vi "2DGraphSetup.vi"(8 "error in (no error)":errorcluster caption="entrée d'erreur (pas d'erreur)", 11 "Interface en entrée":refnum<class "Interface.lvclass"> caption="DNL_LabVIEW Object in") -> (0 "error out":errorcluster caption="sortie d'erreur", 3 "Interface en sortie":refnum<class "Interface.lvclass"> caption="DNL_LabVIEW Object out")   [LabVIEW 2019, in "Interface.lvclass"]
uses:
  Interface.lvclass
  Interface.lvclass/Interface.ctl
  <userlib>/GenProg/ArrayTo1DString.vi
  Experiment Class/Experiment.lvclass
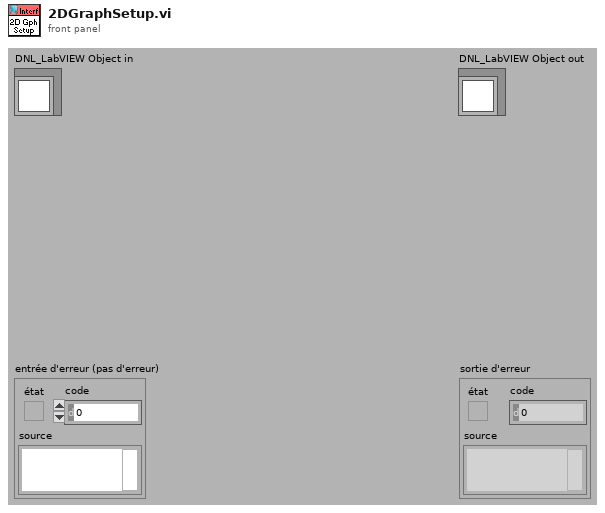
[diagram p1: front panel]
types:
  T1 = typedef "2DGraphSetup.ctl" = cluster{"ZDataIndex":i32, "XParIndex":i32, "YParIndex":i32, "FillLineFirst":bool, "2DGraphIndex":i32, "XParQ Ref":refnum<queue>, "YParQ Ref":refnum<queue>, "DataQRefs":refnum<queue>[], "CurveName":string, "XparInstrInd":i32, "YparInstrInd":i32, "Active":bool}
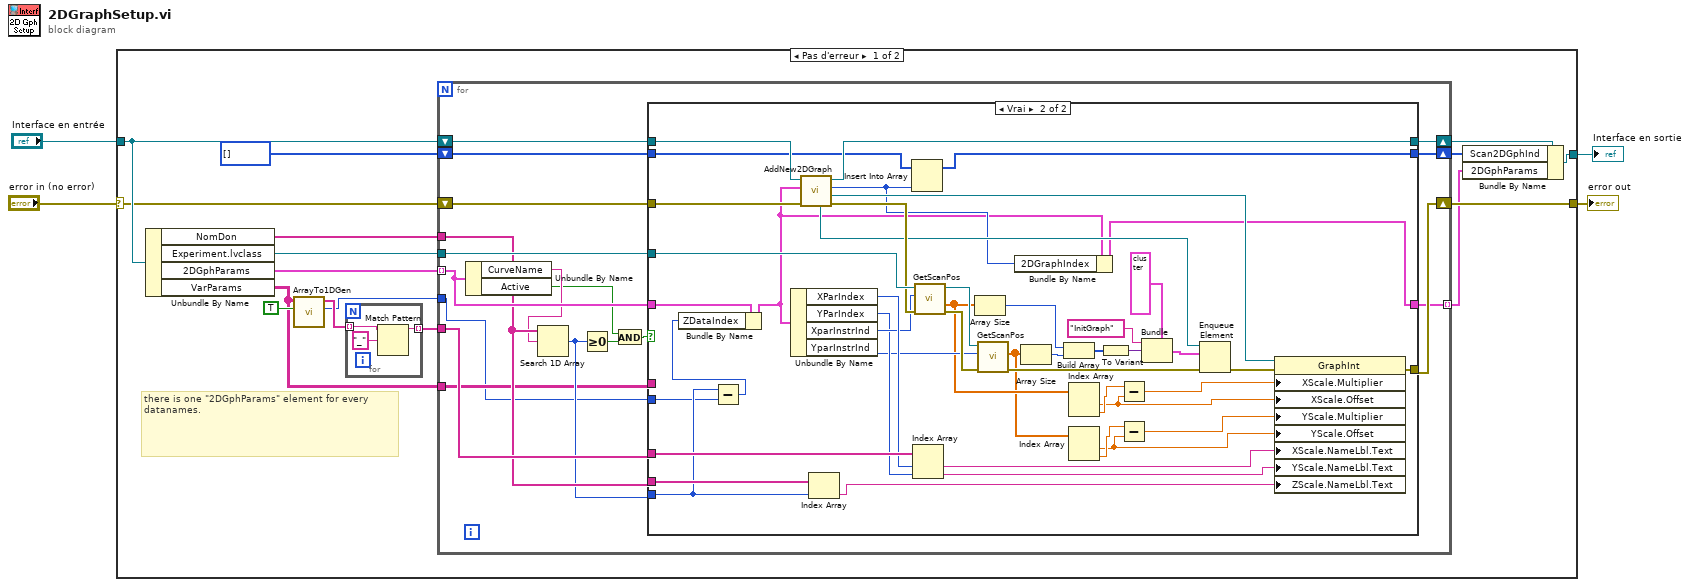
[diagram p0: block diagram]
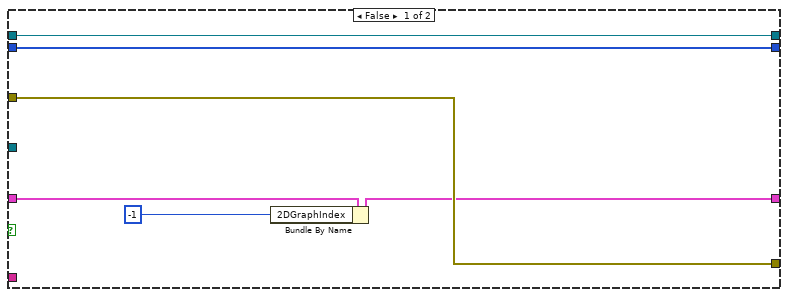
[diagram p2: hidden frame]
diagram:
  n1 = case shown="Pas d'erreur" "error in (no error)" {
    selector: "error in (no error)" -> [w14 w94]
    tunnel: [w12 w94] -> w3
    tunnel: [w17 w93] -> w1
    tunnel: "Interface en entrée" -> [w20 w93]
    frame No Error {
      # "there is one \"2DGphParams\" element for every datanames."
      n2 = Unbundle By Name(w20) -> ("NomDon"=w9:string[], "Experiment.lvclass"=w19:refnum<class "Experiment.lvclass">, "2DGphParams"=w13:T1[], "VarParams"=w7:string[][])
      n3 = call-poly <userlib>:"ArrayTo1DGen.vi"("DelArrEnd"=TRUE, "tableau"=w7) -> ("Size"=w5:i32, "Array Out"=w8:string[])  [unwired: 7 in, 1 out]
      n4 = for {
        tunnel: w8 -> [w23] mode=indexing
        tunnel: [w22] -> w10 mode=indexing
        n5 = Match Pattern(string=w23, regular expression="_" ("expression régulière")) -> (before substring=w22:string)  [unwired: 1 in, 3 out]
      }
      n6 = for {
        tunnel: w13 -> [w41] mode=indexing
        shift-right: [w39] -> w18
        shift-left: w20 -> [w40]
        tunnel: w19 -> [w38]
        shift-right: [w37] -> w16
        shift-left: i32[] [] -> [w36]
        shift-right: [w35] -> w12
        shift-left: w14 -> [w34]
        tunnel: w10 -> [w33]
        tunnel: w9 -> [w32]
        tunnel: w7 -> [w29]
        tunnel: [w25] -> w6 mode=indexing
        tunnel: w5 -> [w24]
        n7 = Unbundle By Name(w41) -> ("CurveName"=w31:string, "Active"=w26:bool)
        n8 = Search 1D Array(1D array=w32, element=w31) -> (index of element=w30:i32)  [unwired: 1 in]
        n9 = Greater Or Equal To 0?(x=w30) -> (x >= 0?=w27:bool)
        n10 = And(x=w26, y=w27) -> (x .and. y?=w28:bool)
        n11 = case shown="Vrai" w28 {
          tunnel: w41 -> [w44 w54]
          tunnel: w40 -> [w47 w92]
          tunnel: [w47 w91] -> w39
          tunnel: w38 -> [_ w88]
          tunnel: [w46 w90] -> w37
          tunnel: w36 -> [w46 w89]
          tunnel: [w45 w73] -> w35
          tunnel: w34 -> [w45 w72]
          tunnel: w33 -> [_ w69]
          tunnel: w32 -> [_ w65]
          tunnel: w30 -> [_ w50]
          tunnel: w29 -> [_ _]
          tunnel: [w43 w53] -> w25
          tunnel: w24 -> [_ w49]
          frame False {
            n12 = Bundle By Name(cluster=w44, "2DGraphIndex"=-1) -> (w43:T1)
          }
          frame True {
            n13 = Subtract(x=w50, y=w49) -> (x-y=w48:i32)
            n14 = Bundle By Name(cluster=w54, "ZDataIndex"=w48) -> (w51:T1)
            n15 = Unbundle By Name(w51) -> ("XParIndex"=w67:i32, "YParIndex"=w62:i32, "XparInstrInd"=w63:i32, "YparInstrInd"=w61:i32)
            n16 = call "AddNew2DGraph.vi"("error in (no error)"=w72, "2DGphParam"=w51, "Interface en entrée"=w92) -> ("error out"=w71:errorcluster, "Graph"=w87:refnum<vi>, "NewGraphInd"=w52:i32, "Interface en sortie"=w91:refnum<class "Interface.lvclass">, "2DGraphQRef"=w70:refnum<queue>)  [unwired: 4 in]
            n17 = Index Array(array=w65, index=w50) -> (element=w64:string)
            n18 = Insert Into Array(array=w89, new element=w52) -> (w90:i32[])  [unwired: 1 in]
            n19 = Index Array(array=w69, index #1=w67, index #2=w62) -> (element #1=w68:string, element #2=w66:string)
            n20 = call "GetScanPos.vi"("error in (no error)"=w71, "ParIndex"=w63, "Experiment en entrée"=w88) -> ("error out"=w83:errorcluster, "ScanTable"=w56:dbl[], "Experiment en sortie"=w84:refnum<class "Experiment.lvclass">)  [unwired: 6 in]
            n21 = Array Size(array=w56) -> (size(s)=w86:i32)
            n22 = call "GetScanPos.vi"("error in (no error)"=w83, "ParIndex"=w61, "Experiment en entrée"=w84) -> ("error out"=w81:errorcluster, "ScanTable"=w55:dbl[])  [unwired: 6 in, 1 out]
            n23 = Bundle By Name(cluster=w51, "2DGraphIndex"=w52) -> (w53:T1)
            n24 = Array Size(array=w55) -> (size(s)=w85:i32)
            n25 = Build Array(w86, w85) -> (w78:i32[])
            n26 = Index Array(array=w56) -> (element #1=w59:dbl, element #2=w60:dbl)  [unwired: 2 in]
            n27 = Index Array(array=w55) -> (element #1=w57:dbl, element #2=w58:dbl)  [unwired: 2 in]
            n28 = To Variant(anything=w78) -> (Variant=w77:variant)
            n29 = Subtract(x=w60, y=w59) -> (x-y=w75:dbl)
            n30 = Subtract(x=w58, y=w57) -> (x-y=w74:dbl)
            n31 = Bundle(cluster=cluster{"Message":string, "Data":variant, i32} {"Message"="", "Data"=variant, 0} ("élément"), "Message"="InitGraph", "Data"=w77) -> (w80:cluster{"Message":string, "Data":variant, i32})  [unwired: 1 in]
            n32 = Enqueue Element(queue=w70, element=w80, error in (no error)=w81) -> (error out=w76:errorcluster)  [unwired: 1 in, 2 out]
            n33 = property class="GraphInt"(reference=w87, error in=w76, "XScale.Multiplier"=w75, "XScale.Offset"=w59, "YScale.Multiplier"=w74, "YScale.Offset"=w57, "XScale.NameLbl.Text"=w68, "YScale.NameLbl.Text"=w66, "ZScale.NameLbl.Text"=w64) -> (error out=w73:errorcluster)  [unwired: 1 out]
          }
        }
      }
      n34 = Bundle By Name(cluster=w18, "Scan2DGphInd"=w16, "2DGphParams"=w6) -> (w17:refnum<class "Interface.lvclass">)
    }
    frame Error {
    }
  }
  "error out" <- w3
  "Interface en sortie" <- w1
